vi "OpenVIReference_RCM.vi"(8 "error in (no error)":errorcluster, 11 "path":path) -> (0 "error out":errorcluster, 3 "vi reference":refnum<vi>)   [LabVIEW 2009, in "RCM.xctl"]
uses:
  RCM.xctl
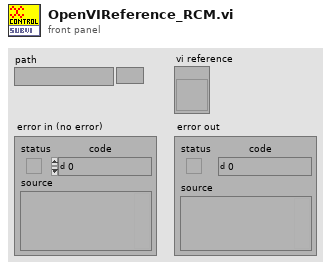
[diagram p1: front panel]
types:
  T1 = enum32{"Invalid", "Standard", "Closed", "Hidden", "Minimized", "Maximized"}
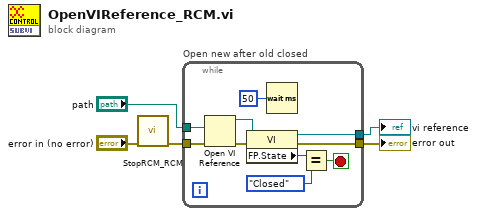
[diagram p0: block diagram]
diagram:
  n1 = call "StopRCM_RCM.vi"("error in (no error)"="error in (no error)") -> ("error out"=w3:errorcluster)  [unwired: 13 in, 1 out]
  n2 = while "Open new after old closed" {
    tunnel: w3 -> [w15]
    tunnel: "path" -> [w13]
    tunnel: [w12] -> w5
    tunnel: [w6] -> w1
    stop <- w7 stop-if-true
    n3 = Open VI Reference(vi path=w13, error in (no error)=w15) -> (vi reference=w10:refnum<vi>, error out=w11:errorcluster)  [unwired: 4 in]
    n4 = property class="VI"(reference=w10, error in=w11) -> (reference out=w12:refnum<vi>, error out=w6:errorcluster, "FP.State"=w9:T1)
    n5 = Wait (ms)(milliseconds to wait=u32 50) -> ()  [unwired: 1 out]
    n6 = Equal?(x=w9, y=T1."Closed") -> (x = y?=w7:bool)
  }
  "vi reference" <- w5
  "error out" <- w1
